vi "Configuration Dialog.vi"(8 "error in (no error)":errorcluster, 11 "Report Generator In":refnum<class "Report Generator.lvclass">) -> (0 "error out":errorcluster, 3 "Report Generator Out":refnum<class "Report Generator.lvclass">)   [LabVIEW 2020, in "Report Generator.lvclass"]
uses:
  Report Generator.lvclass
  Report Classes/Test Report/Test Report.lvclass
panel:
  in  "Group by date?":bool
  in  "Report Name":string
  in  "Auto-generate report?":bool
  in  "Report Type":u16(ring) items=["Plain Text Report", "XML Report"]
  in  "Report Directory Path":path
  in  "Cancel":bool
  in  "Commit":bool
  in  "Open when saved":bool
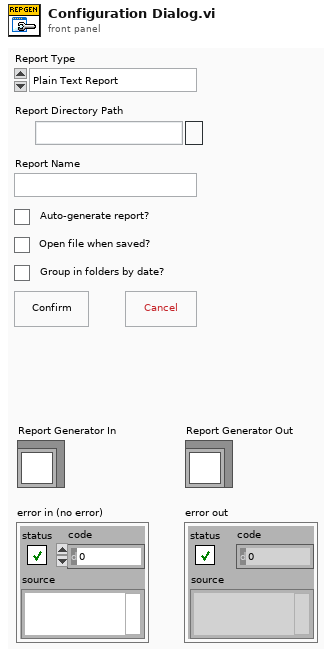
[diagram p1: front panel]
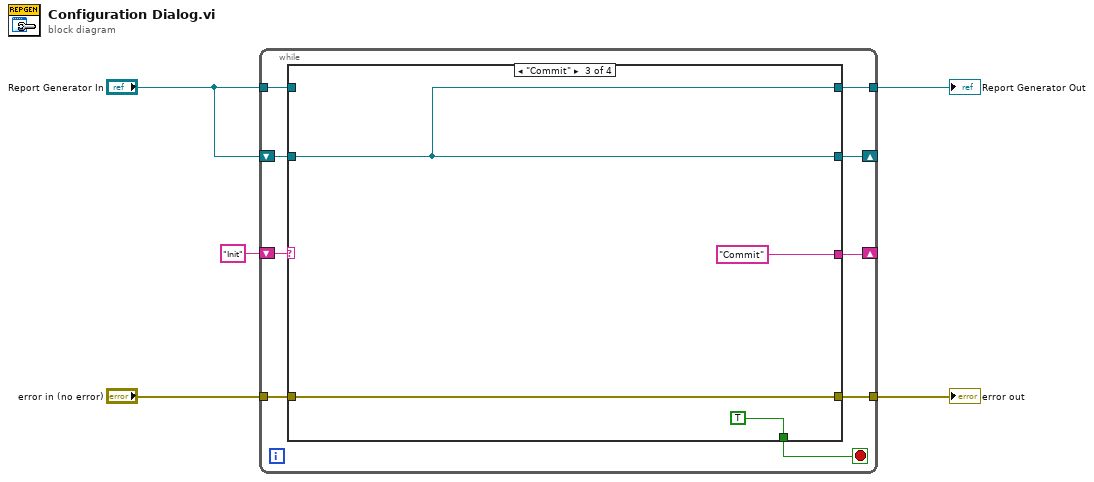
[diagram p0: block diagram]
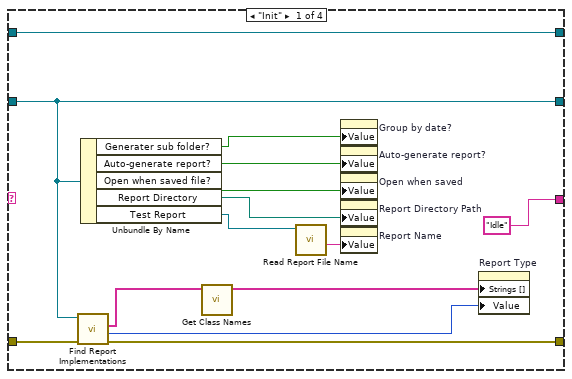
[diagram p2: hidden frame]
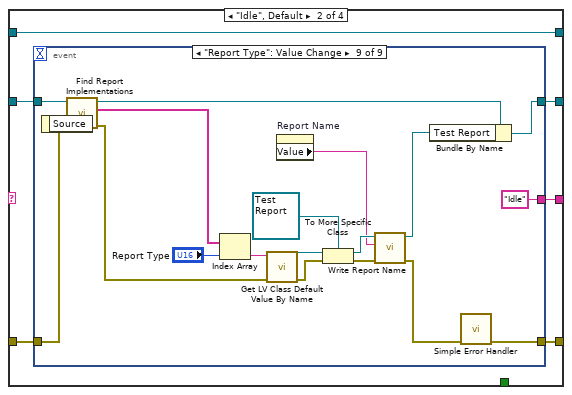
[diagram p3: hidden frame]
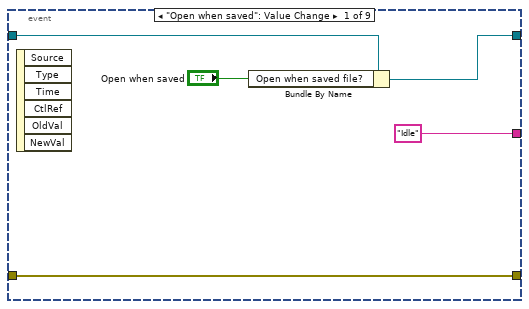
[diagram p4: hidden frame]
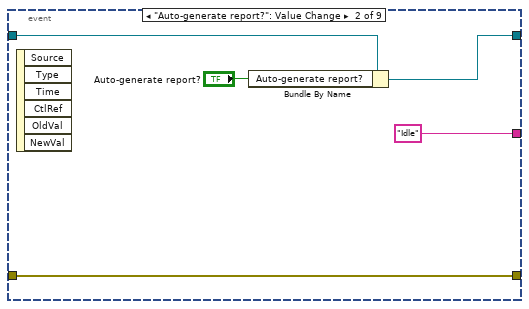
[diagram p5: hidden frame]
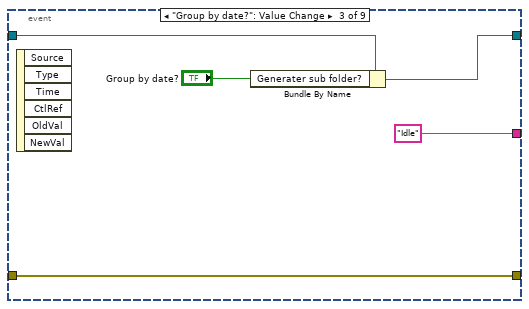
[diagram p6: hidden frame]
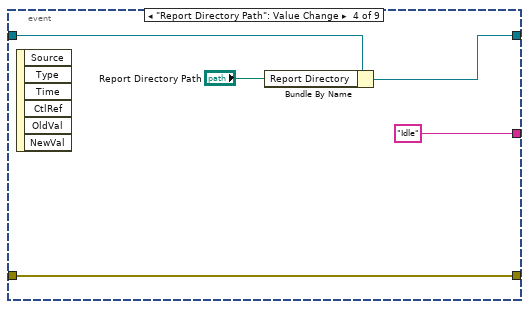
[diagram p7: hidden frame]
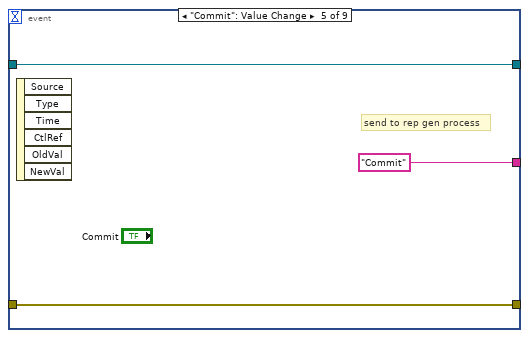
[diagram p8: hidden frame]
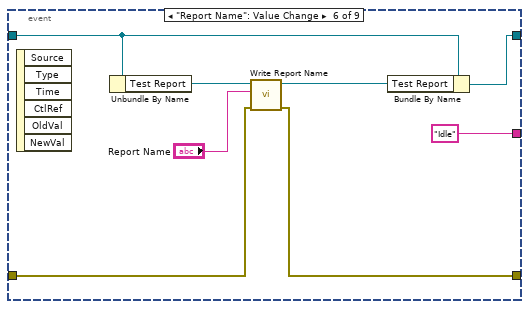
[diagram p9: hidden frame]
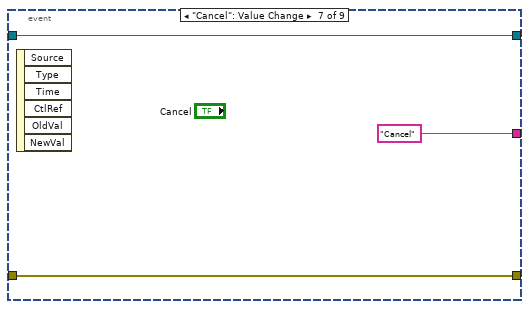
[diagram p10: hidden frame]
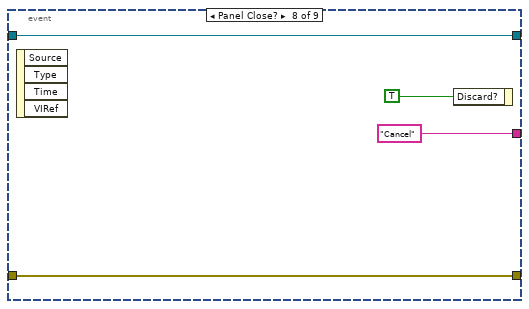
[diagram p11: hidden frame]
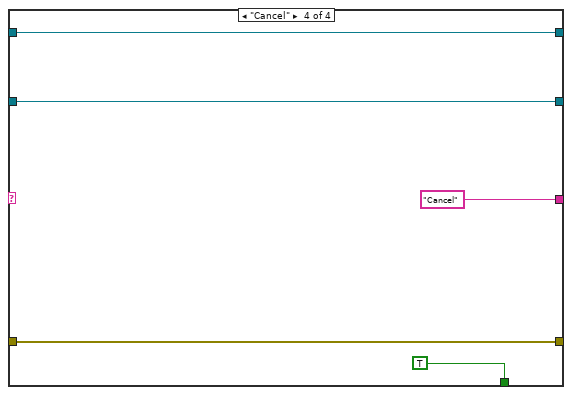
[diagram p12: hidden frame]
diagram:
  n1 = while {
    tunnel: [w14] -> w5
    tunnel: "Report Generator In" -> [w13]
    tunnel: [w12] -> w4
    tunnel: "error in (no error)" -> [w11]
    shift-right: [w8] -> _
    shift-left: "Report Generator In" -> [w9]
    shift-right: [w6] -> _
    shift-left: "Init" -> [w7]
    stop <- w10 stop-if-true
    n2 = case shown="\"Commit\"" w7 {
      tunnel: [w28 w30 w94 w99] -> w14
      tunnel: w13 -> [w28 w30 _ w99]
      tunnel: [w24 w34 w93 w95] -> w12
      tunnel: w11 -> [w23 w33 w93 w95]
      tunnel: [_ _ TRUE TRUE] -> w10
      tunnel: w9 -> [w22 w32 w94 w98]
      tunnel: [w22 w31 w94 w98] -> w8
      tunnel: ["Idle" w29 "Commit" "Cancel"] -> w6
      frame "Init" {
        n3 = call "Find Report Implementations.vi"("error in (no error)"=w23, "Report Generator In"=w22) -> ("error out"=w24:errorcluster, "Active index"=w21:i32, "Test Reports"=w16:string[])  [unwired: 6 in, 1 out]
        n4 = Unbundle By Name(w22) -> ("Generater sub folder?"=w17:bool, "Auto-generate report?"=w18:bool, "Open when saved file?"=w26:bool, "Report Directory"=w25:path, "Test Report"=w20:refnum<class "Test Report.lvclass">)
        n5 = call "Get Class Names.vi"("Qualified names"=w16) -> ("Class names only"=w15:string[])  [unwired: 10 in]
        n6 = call-dynamic "Read Report File Name.vi"("Report In"=w20) -> ("Report File Name without extension"=w19:string)  [unwired: 7 in, 3 out]
        n7 = property on="Group by date?" class="Bool (strict)"("Value"=w17) -> ()  [unwired: 2 in, 2 out]
        n8 = property on="Auto-generate report?" class="Bool (strict)"("Value"=w18) -> ()  [unwired: 2 in, 2 out]
        n9 = property on="Open when saved" class="Bool (strict)"("Value"=w26) -> ()  [unwired: 2 in, 2 out]
        n10 = property on="Report Directory Path" class="Path"("Value"=w25) -> ()  [unwired: 2 in, 2 out]
        n11 = property on="Report Name" class="Str"("Value"=w19) -> ()  [unwired: 2 in, 2 out]
        n12 = property on="Report Type" class="Ring (strict)"("Strings []"=w15, "Value"=w21) -> ()  [unwired: 2 in, 2 out]
      }
      frame "Idle", Default {
        n13 = event shown="[8] \"Report Type\": Value Change" {
          selector: _ -> [_ _ _ _ _ _ _ _ _]
          dyn-events: _ -> [_ _ _ _ _ _ _ _ _]
          timeout: _ -> [_ _ _ _ _ _ _ _ _]
          tunnel: [w39 w44 w49 w54 w56 w59 w68 w72 w73] -> w34
          tunnel: w33 -> [w39 w44 w49 w54 w56 w58 w68 w72 w74]
          tunnel: w32 -> [w38 w43 w48 w53 w57 w63 w67 w71 w78]
          tunnel: [w37 w42 w47 w52 w57 w64 w67 w71 w88] -> w31
          tunnel: ["Idle" "Idle" "Idle" "Idle" "Commit" "Idle" "Cancel" "Cancel" "Idle"] -> w29
          event "Open when saved": Value Change {
            n14 = event-data() -> ()  [unwired: 1 in, 6 out]
            n15 = Bundle By Name(cluster=w38, "Open when saved file?"="Open when saved") -> (w37:refnum<class "Report Generator.lvclass">)
          }
          event "Auto-generate report?": Value Change {
            n16 = event-data() -> ()  [unwired: 1 in, 6 out]
            n17 = Bundle By Name(cluster=w43, "Auto-generate report?"="Auto-generate report?") -> (w42:refnum<class "Report Generator.lvclass">)
          }
          event "Group by date?": Value Change {
            n18 = event-data() -> ()  [unwired: 1 in, 6 out]
            n19 = Bundle By Name(cluster=w48, "Generater sub folder?"="Group by date?") -> (w47:refnum<class "Report Generator.lvclass">)
          }
          event "Report Directory Path": Value Change {
            n20 = event-data() -> ()  [unwired: 1 in, 6 out]
            n21 = Bundle By Name(cluster=w53, "Report Directory"="Report Directory Path") -> (w52:refnum<class "Report Generator.lvclass">)
          }
          event "Commit": Value Change {
            # "send to rep gen process"
            n22 = event-data() -> ()  [unwired: 1 in, 6 out]
          }
          event "Report Name": Value Change {
            n23 = event-data() -> ()  [unwired: 1 in, 6 out]
            n24 = Unbundle By Name(w63) -> ("Test Report"=w62:refnum<class "Test Report.lvclass">)
            n25 = call "Write Report Name.vi"("error in (no error)"=w58, "Report Name"="Report Name", "Report In"=w62) -> ("error out"=w59:errorcluster, "Report Out"=w60:refnum<class "Test Report.lvclass">)  [unwired: 7 in]
            n26 = Bundle By Name(cluster=w63, "Test Report"=w60) -> (w64:refnum<class "Report Generator.lvclass">)
          }
          event "Cancel": Value Change {
            n27 = event-data() -> ()  [unwired: 1 in, 6 out]
          }
          event Panel Close? {
            n28 = event-data() -> ()  [unwired: 1 in, 4 out]
            n29 = event-data("Discard?"=TRUE) -> ()  [unwired: 1 in, 1 out]
          }
          event "Report Type": Value Change {
            n30 = event-data() -> ()  [unwired: 1 in, 1 out]
            n31 = call "Find Report Implementations.vi"("error in (no error)"=w74, "Report Generator In"=w78) -> ("error out"=w75:errorcluster, "Test Reports"=w77:string[], "Report Generator Out"=w79:refnum<class "Report Generator.lvclass">)  [unwired: 6 in, 1 out]
            n32 = Index Array(array=w77, index="Report Type") -> (element=w76:string)
            n33 = call <vilib>:"Get LV Class Default Value By Name.vi"("error in (no error)"=w75, "class name"=w76) -> ("error out"=w85:errorcluster, "object"=w87:refnum<class>)  [unwired: 8 in]
            n34 = property on="Report Name" class="Str"() -> ("Value"=w82:string)  [unwired: 2 in, 2 out]
            n35 = To More Specific Class(target class=refnum<class "Test Report.lvclass"> refnum ("Test Report"), reference=w87, error in=w85) -> (specific class reference=w84:refnum<class "Test Report.lvclass">, error out=w81:errorcluster)
            n36 = call "Write Report Name.vi"("error in (no error)"=w81, "Report Name"=w82, "Report In"=w84) -> ("error out"=w80:errorcluster, "Report Out"=w83:refnum<class "Test Report.lvclass">)  [unwired: 7 in]
            n37 = Bundle By Name(cluster=w79, "Test Report"=w83) -> (w88:refnum<class "Report Generator.lvclass">)
            n38 = call <vilib>:"Simple Error Handler.vi"("error in (no error)"=w80) -> ("error out"=w73:errorcluster)  [unwired: 4 in, 4 out]
          }
        }
      }
      frame "Commit" {
      }
      frame "Cancel" {
      }
    }
  }
  "error out" <- w4
  "Report Generator Out" <- w5
